vi "XRS450 SPI Gyro.vi"() -> ()   [LabVIEW 2015]
doc: "XRS450 SPI Gyro Example\n\nThis example shows how to use the Analog Devices XRS450 gyro connected to the SPI port on the RoboRIO.\n\nThis example expects a USB cable connected from your development PC to the Type B USB Jack (next to the power input) on the roboRIO.\n\nThis example expects the Driver Station to be running."
uses:
  <vilib>/Rock Robotics/SystemInterfaces/spilib/spi_bus.ctl
  <vilib>/Rock Robotics/WPI/Gyro/WPI_GyroXRS450_SPI_Open.vi
panel:
  out "Calibrated?":bool
  in  "Reset Angle?":bool
  out "Device Found":bool
  in  "stop":bool
  out "Angle":dbl(knob) scale=0.0..360.0
  in  "SPI Bus":T1
  in  "Sample Rate (ms)":dbl=1.0 min=0.0 max=100.0 step=0.25 format="%#_13g"
  # "Set these inputs before running."
  # "This can be set while running."
  # "This will display the current gyro angle."
  # "This shows wiring for the Analog Devices XRS450 gyro.  It can be plugged directly into the SPI port."
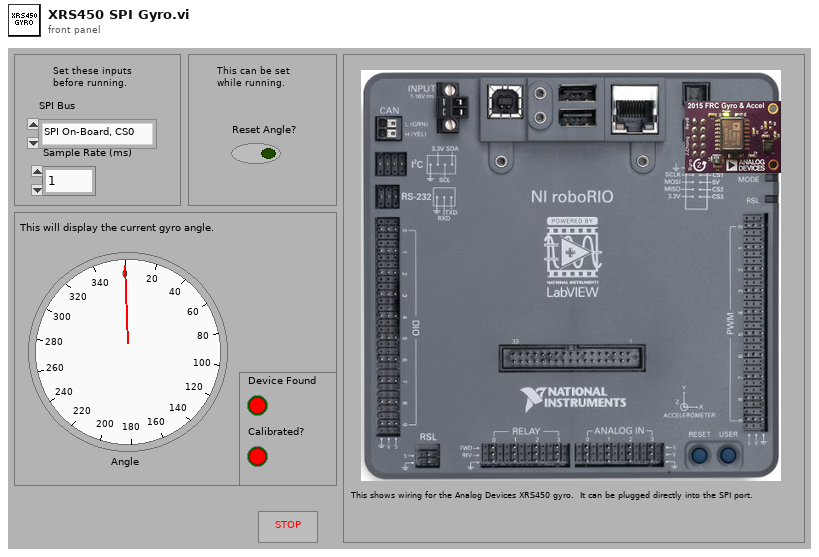
[diagram p1: front panel]
types:
  T1 = typedef "spi_bus.ctl" = enum16{"SPI On-Board, CS0", "SPI On-Board, CS1", "SPI On-Board, CS2", "SPI On-Board, CS3", "SPI MXP", "Invalid"}
  T2 = typedef "WPI_GyroDevRef.ctl" = cluster{"DevStatus":errorcluster, "Analog Channel":T3, "Offset":dbl, "Gain (VoltsPerDegree/Second)":dbl, "Gyro Type":enum16{"Analog", "XRS450"}, "Handle":i32, "SPI Bus":T1, "Device Found":bool, "Sample Rate":dbl, "Calibrate On Open":bool}
  T3 = typedef "FPGA_AIChannel.ctl" = enum8{"AI 0", "AI 1", "AI 2", "AI 3", "AI MXP 0", "AI MXP 1", "AI MXP 2", "AI MXP 3", "Invalid"}
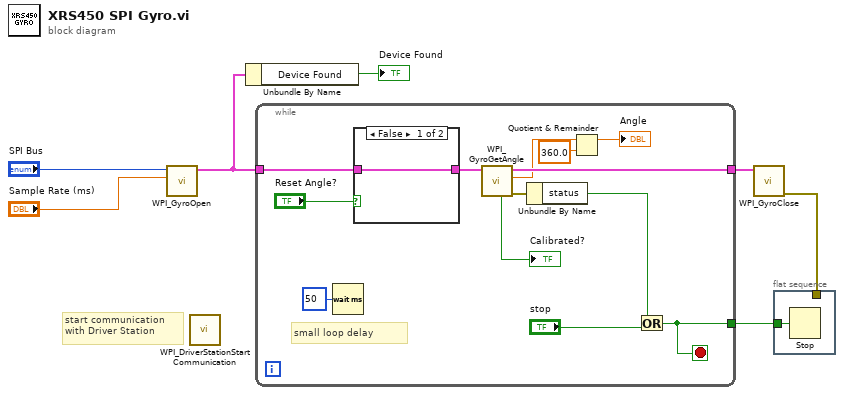
[diagram p0: block diagram]
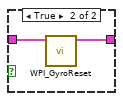
[diagram p2: hidden frame]
diagram:
  # "start communication with Driver Station"
  n1 = call-poly <vilib>:"WPI_GyroOpen.vi"("Sample Rate (ms)"="Sample Rate (ms)", "SPI Bus"="SPI Bus") -> ("GyroDevRef"=w3:T2)  [unwired: 8 in, 1 out]
  n2 = call <vilib>:"WPI_DriverStationStart Communication.vi"() -> ()  [unwired: 12 in]
  n3 = Unbundle By Name(w3) -> ("Device Found"=→"Device Found":bool)
  n4 = while {
    tunnel: w3 -> [w16]
    tunnel: [w13] -> w5
    tunnel: [w11] -> w6
    stop <- w13 stop-if-true
    # "small loop delay"
    n5 = Wait (ms)(milliseconds to wait=u32 50) -> ()  [unwired: 1 out]
    n6 = case shown="False" "Reset Angle?" {
      tunnel: w16 -> [w21 w23]
      tunnel: [w21 w22] -> w12
      frame False {
      }
      frame True {
        n7 = call <vilib>:"WPI_GyroReset.vi"("GyroDevRef"=w23) -> ("GyroDevRef"=w22:T2)  [unwired: 9 in, 1 out]
      }
    }
    n8 = call <vilib>:"WPI_GyroGetAngle.vi"("GyroDevRef"=w12) -> ("error out"=w9:errorcluster, "Angle"=w10:dbl, "GyroDevRef"=w11:T2, "Calibrated?"=→"Calibrated?":bool)  [unwired: 6 in, 1 out]
    n9 = Unbundle By Name(w9) -> ("status"=w14:bool)
    n10 = Quotient & Remainder(x=w10, y=360.0) -> (x-y*floor(x/y)=→"Angle":dbl)  [unwired: 1 out]
    n11 = Or(x=w14, y="stop") -> (x .or. y?=w13:bool)
  }
  n12 = call <vilib>:"WPI_GyroClose.vi"("GyroDevRef"=w6) -> ("error out"=w4:errorcluster)  [unwired: 10 in]
  n13 = flat-sequence {
    tunnel: w5 -> [w24]
    tunnel: w4 -> [_]
    frame #0 {
      n14 = Stop(stop? (T)=w24) -> ()
    }
  }
